vi "Idle_Action.vi"(5 "GuiRef":T1={"StringOut"=refnum, "AbortOnFail"=refnum, "SN"=refnum, "SN_Length"=refnum, "TestResult"=refnum, "CycleTime"=refnum, "ErrorCode"=refnum, "UUTStatus"=refnum, "DataBaseEnable?"=refnum, "DUTModel"=refnum, "FixtureID"=refnum, "OperatorID"=refnum, "SNReady"=refnum, "StopSlot"=refnum, "NextStep"=refnum, "PassYeild"=refnum, "Failed"=refnum, "Passed"=refnum, "Tested"=refnum, "TestItemsCtl"={"StepName"="", "TestEnable"=FALSE, "LoopCount"=0, "StopOnFail"=FALSE, "Index"=0, "TestName"="", "通道"="", "参数"="", "TimeStart"=0}, "ProcessBar"=refnum, "Slot"=enum."Slot1", "Row"=3, "States"=refnum, "TestMode"=refnum, "循环次数-DUT"=refnum, "波形图"=refnum, "产品型号"=refnum, "子面板"=refnum, "测试失败项目"=refnum, "测试结果"=refnum, "DUT"=refnum, "Starttime"=refnum, "SlotReady"=refnum, "版本信息"=refnum, "WIFI_1"=refnum, "WIFI_2"=refnum, "直通率"=refnum, "卡1开卡结果"=refnum, "卡2开卡结果"=refnum}, 7 "Slot":T3, 8 "error in":errorcluster, 9 "SNReady":refnum<vi>, 11 "SlotEnable":refnum<vi>) -> (0 "error out":errorcluster, 3 "SlotReady":bool)   [LabVIEW 2013]
uses:
  SystemCode/SysControl/Slot.ctl
  SystemCode/SysControl/Reference.ctl
  SystemCode/SysControl/TestItemsCTL.ctl
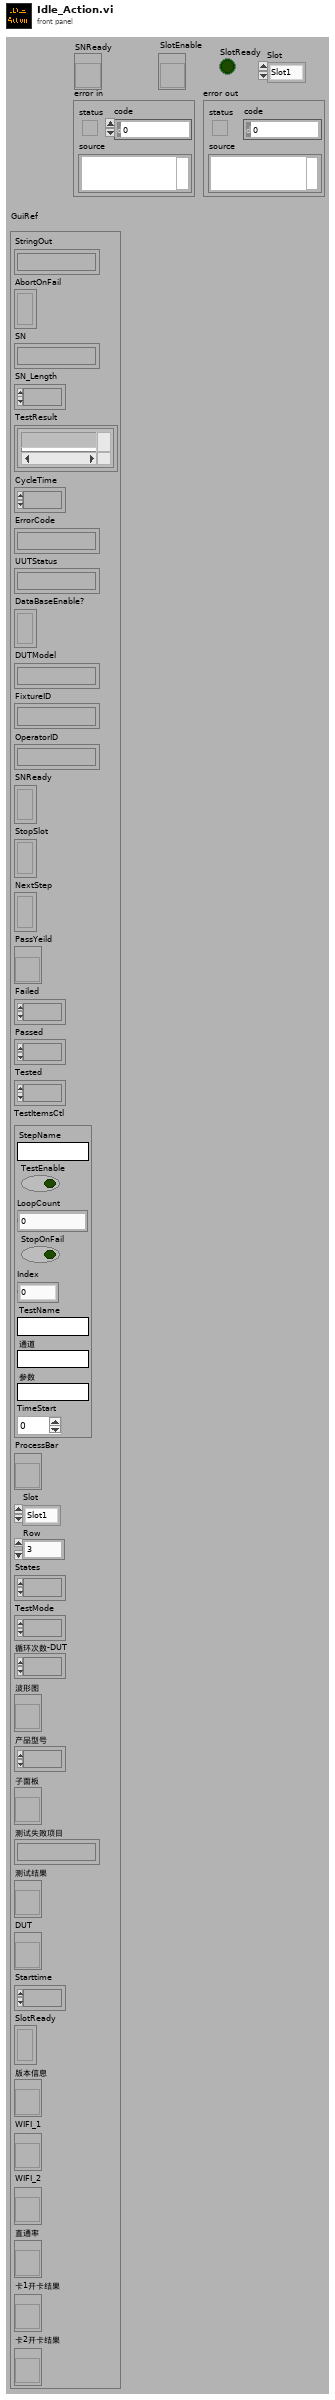
[diagram p1: front panel]
types:
  T1 = typedef "Reference.ctl" = cluster{"StringOut":refnum<vi>, "AbortOnFail":refnum<vi>, "SN":refnum<vi>, "SN_Length":refnum<vi>, "TestResult":refnum<vi>, "CycleTime":refnum<vi>, "ErrorCode":refnum<vi>, "UUTStatus":refnum<vi>, "DataBaseEnable?":refnum<vi>, "DUTModel":refnum<vi>, "FixtureID":refnum<vi>, "OperatorID":refnum<vi>, "SNReady":refnum<vi>, "StopSlot":refnum<vi>, "NextStep":refnum<vi>, "PassYeild":refnum<vi>, "Failed":refnum<vi>, "Passed":refnum<vi>, "Tested":refnum<vi>, "TestItemsCtl":T2, "ProcessBar":refnum<vi>, "Slot":T3, "Row":u32, "States":refnum<vi>, "TestMode":refnum<vi>, "循环次数-DUT":refnum<vi>, "波形图":refnum<vi>, "产品型号":refnum<vi>, "子面板":refnum<vi>, "测试失败项目":refnum<vi>, "测试结果":refnum<vi>, "DUT":refnum<vi>, "Starttime":refnum<vi>, "SlotReady":refnum<vi>, "版本信息":refnum<vi>, "WIFI_1":refnum<vi>, "WIFI_2":refnum<vi>, "直通率":refnum<vi>, "卡1开卡结果":refnum<vi>, "卡2开卡结果":refnum<vi>}
  T2 = typedef "TestItemsCTL.ctl" = cluster{"StepName":string, "TestEnable":bool, "LoopCount":i32, "StopOnFail":bool, "Index":u32, "TestName":string, "通道":string, "参数":string, "TimeStart":u32}
  T3 = typedef "Slot.ctl" = enum16{"Slot1", "Slot2", "Slot3", "Slot4"}
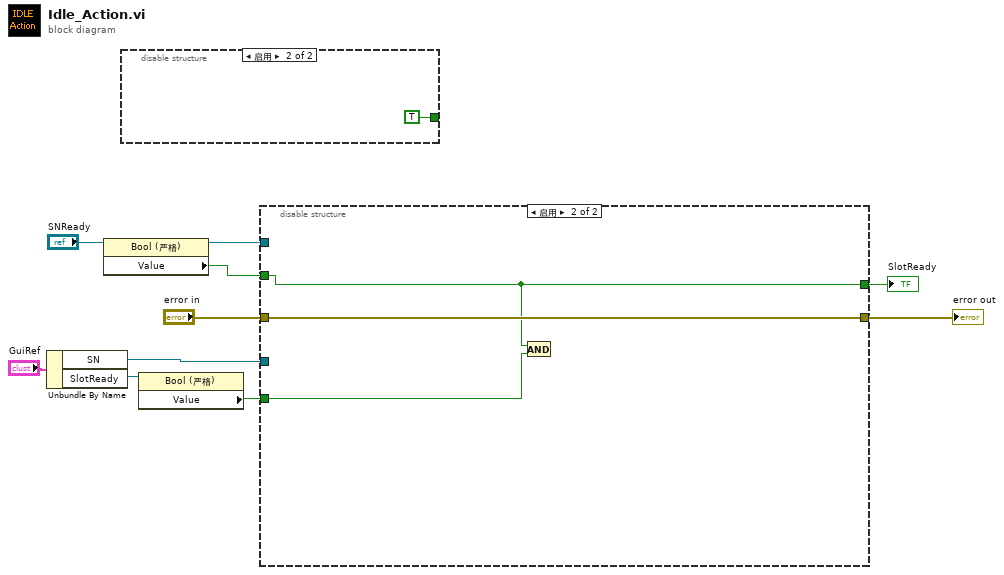
[diagram p0: block diagram]
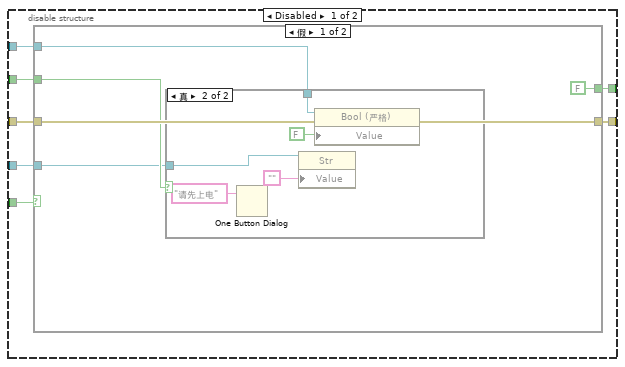
[diagram p2: hidden frame]
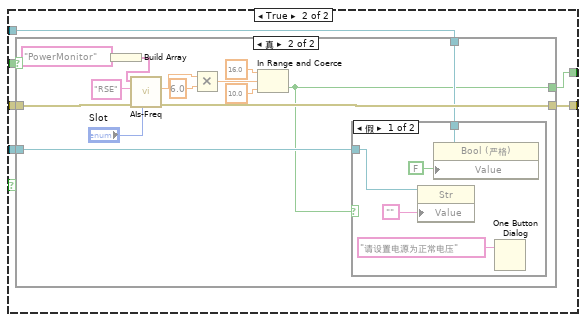
[diagram p4: hidden frame]
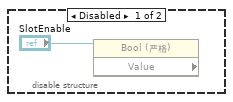
[diagram p7: hidden frame]
diagram:
  n1 = Unbundle By Name("GuiRef") -> ("SN"=w4:refnum<vi>, "SlotReady"=w2:refnum<vi>)
  n2 = property class="Bool (严格)"(reference="SNReady") -> (reference out=w3:refnum<vi>, "Value"=w9:bool)  [unwired: 1 in, 1 out]
  n3 = disable-structure shown="启用" {
    disable-tunnel: [_ TRUE ("x")] -> _
    frame Disabled {
      n4 = property class="Bool (严格)" props=["Value"](reference="SlotEnable") -> ()  [unwired: 1 in, 3 out]
    }
    frame Enabled {
    }
  }
  n5 = property class="Bool (严格)"(reference=w2) -> ("Value"=w1:bool)  [unwired: 1 in, 2 out]
  n6 = disable-structure shown="启用" {
    disable-tunnel: w9 -> [w19 w56]
    disable-tunnel: "error in" -> [w18 w58]
    disable-tunnel: [w17 w58] -> w7
    disable-tunnel: [w16 w56] -> w6
    disable-tunnel: w4 -> [w15 _]
    disable-tunnel: w3 -> [w14 _]
    disable-tunnel: w1 -> [w13 w57]
    frame Disabled {
      n7 = case shown="假" w13 {
        tunnel: w19 -> [w22 w35]
        tunnel: w18 -> [w23 w34]
        tunnel: [w23 w33] -> w17
        tunnel: [FALSE w32] -> w16
        tunnel: w15 -> [w20 w31]
        tunnel: w14 -> [w21 w30]
        frame False {
          n8 = case shown="真" w22 {
            tunnel: w21 -> [_ w26]
            tunnel: w20 -> [_ w25]
            frame False {
            }
            frame True {
              n9 = One Button Dialog(message="请先上电" ("消息")) -> ()  [unwired: 1 in, 1 out]
              n10 = property class="Str"(reference=w25, "Value"="") -> ()  [unwired: 1 in, 2 out]
              n11 = property class="Bool (严格)"(reference=w26, "Value"=FALSE ("值")) -> ()  [unwired: 1 in, 2 out]
            }
          }
        }
        frame True {
          n12 = case shown="真" w35 {
            tunnel: w34 -> [w36 w45]
            tunnel: [w36 w44] -> w33
            tunnel: [_ w40] -> w32
            tunnel: w31 -> [_ w42]
            tunnel: w30 -> [_ w41]
            frame False {
            }
            frame True {
              n13 = Build Array("PowerMonitor" ("CH")) -> (w38:string[])
              n14 = call "AIs-Freq.vi"("Slot"="Slot", "error in"=w45, "Mode"="RSE", "CHs"=w38) -> ("error out"=w44:errorcluster, "RMS value"=w37:dbl)  [unwired: 5 in, 1 out]
              n15 = Multiply(x=w37, y=6.0) -> (x*y=w49:dbl)
              n16 = In Range and Coerce(upper limit=16.0 ("上限"), x=w49, lower limit=10.0 ("下限")) -> (In Range?=w40:bool)  [unwired: 1 out]
              n17 = case shown="假" w40 {
                tunnel: w42 -> [w54 _]
                tunnel: w41 -> [w52 _]
                frame False {
                  n18 = property class="Str"(reference=w54, "Value"="") -> ()  [unwired: 1 in, 2 out]
                  n19 = property class="Bool (严格)"(reference=w52, "Value"=FALSE ("值")) -> ()  [unwired: 1 in, 2 out]
                  n20 = One Button Dialog(message="请设置电源为正常电压" ("消息")) -> ()  [unwired: 1 in, 1 out]
                }
                frame True {
                }
              }
            }
          }
        }
      }
    }
    frame Enabled {
      n21 = And(x=w56, y=w57) -> ()  [unwired: 1 out]
    }
  }
  "error out" <- w7
  "SlotReady" <- w6
